vi "Split Text Into Words.vi"(11 "VI Name":string) -> (3 "Array":string[](array[string]))   [LabVIEW 2020, in "Text-Based VI Icon.lvlib"]
doc: "Splits Text strings into words.\nThis VI supports splitting based on CamelCase or one of the following delimiters:\n- Space \" \"\n- Underscore \"_\"\n\nExample of use: \"The_VI Name\" -> [\"The\",\"VI\",\"Name\"]"
uses:
  Text-Based VI Icon.lvlib
  <vilib>/regexp/Match Regular Expression.xnode
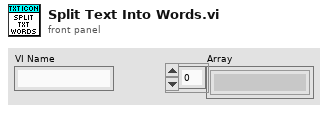
[diagram p1: front panel]
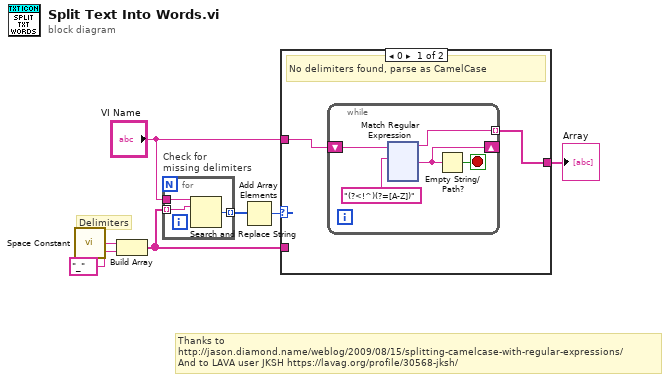
[diagram p0: block diagram]
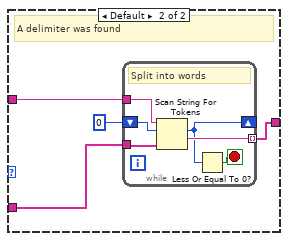
[diagram p2: hidden frame]
diagram:
  # "Delimiters"
  # "Thanks to\nhttp://jason.diamond.name/weblog/2009/08/15/splitting-camelcase-with-regular-expressions/\nAnd to LAVA user JKSH https://lavag.org/profile/30568-jksh/"
  n1 = call <vilib>:"Space Constant.vi"() -> ("String"=w5:string)
  n2 = Build Array(w5, "_") -> (w3:string[])
  n3 = for "Check for \nmissing delimiters" {
    tunnel: [w10] -> w2 mode=indexing
    tunnel: "VI Name" -> [w9]
    tunnel: w3 -> [w8] mode=indexing
    n4 = Search and Replace String(input string=w9, search string=w8) -> (number of replacements=w10:i32)  [unwired: 6 in, 3 out]
  }
  n5 = Add Array Elements(numeric array=w2) -> (sum=w1:i32)
  n6 = case shown="0" w1 {
    tunnel: [w11 w138] -> w7
    tunnel: "VI Name" -> [w12 w136]
    tunnel: w3 -> [_ w135]
    frame 0 {
      # "No delimiters found, parse as CamelCase"
      n7 = while {
        shift-right: [w14] -> _
        shift-left: w12 -> [w15]
        tunnel: [w13] -> w11 mode=indexing
        stop <- w17 stop-if-true
        n8 = xnode "Match Regular Expression"("input string"=w15, "regular expression"="(?<!^)(?=[A-Z])") -> ("before match"=w13:string, "after match"=w14:string)  [unwired: 4 in, 3 out]
        n9 = Empty String/Path?(string/path=w14) -> (empty?=w17:bool)
      }
    }
    frame Default {
      # "A delimiter was found"
      n10 = while {
        tunnel: w136 -> [w144]
        shift-right: [w141] -> _
        shift-left: 0 ("offset past token") -> [w143]
        tunnel: [w142] -> w138 mode=indexing
        tunnel: w135 -> [w139]
        stop <- w140 stop-if-true
        # "Split into words"
        n11 = Scan String For Tokens(6:w139, 8:w143, 9:w144) -> (1:w142:string, 2:w141:i32)  [unwired: 3 in, 2 out]
        n12 = Less Or Equal To 0?(x=w141) -> (x <= 0?=w140:bool)
      }
    }
  }
  "Array" <- w7
